vi "POO 1 - objet.vi"() -> ()   [LabVIEW 2023]
uses:
  Controller/Ctrl_ID.ctl
  Impot/Impot.lvclass
  ID/ID.lvclass
panel:
  in  "Annual ressource":dbl=100.0 format="%#_13g $"
  out "Tax evaluation":dbl
  out "Read ID after reset":T1
  out "Read ID":T1
  in  "Write ID":T1
  # "Write"
  # "Read"
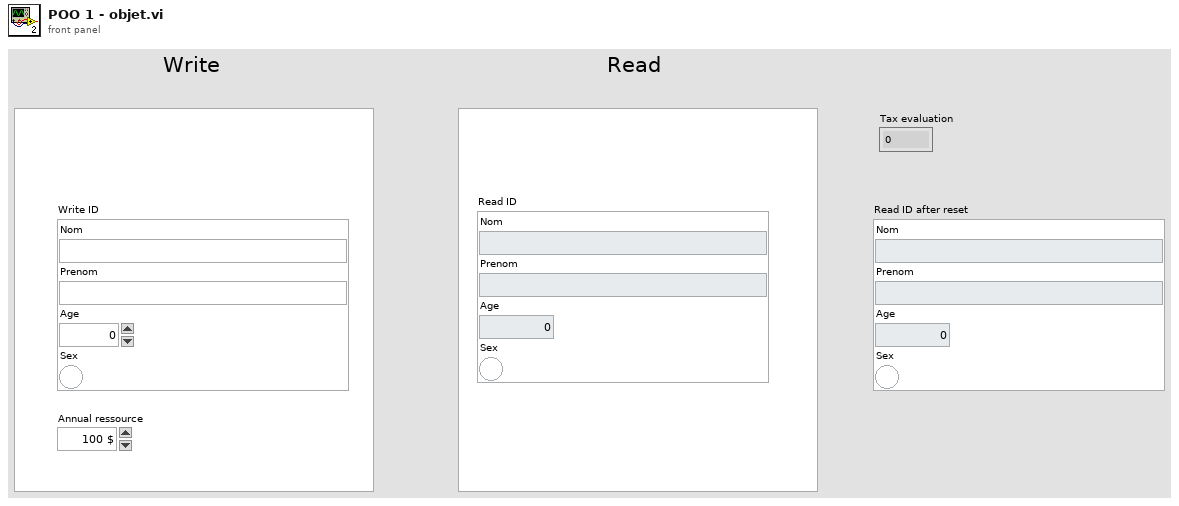
[diagram p1: front panel]
types:
  T1 = typedef "Ctrl_ID.ctl" = cluster{"Nom":string, "Prenom":string, "Age":u8, "Sex":bool}
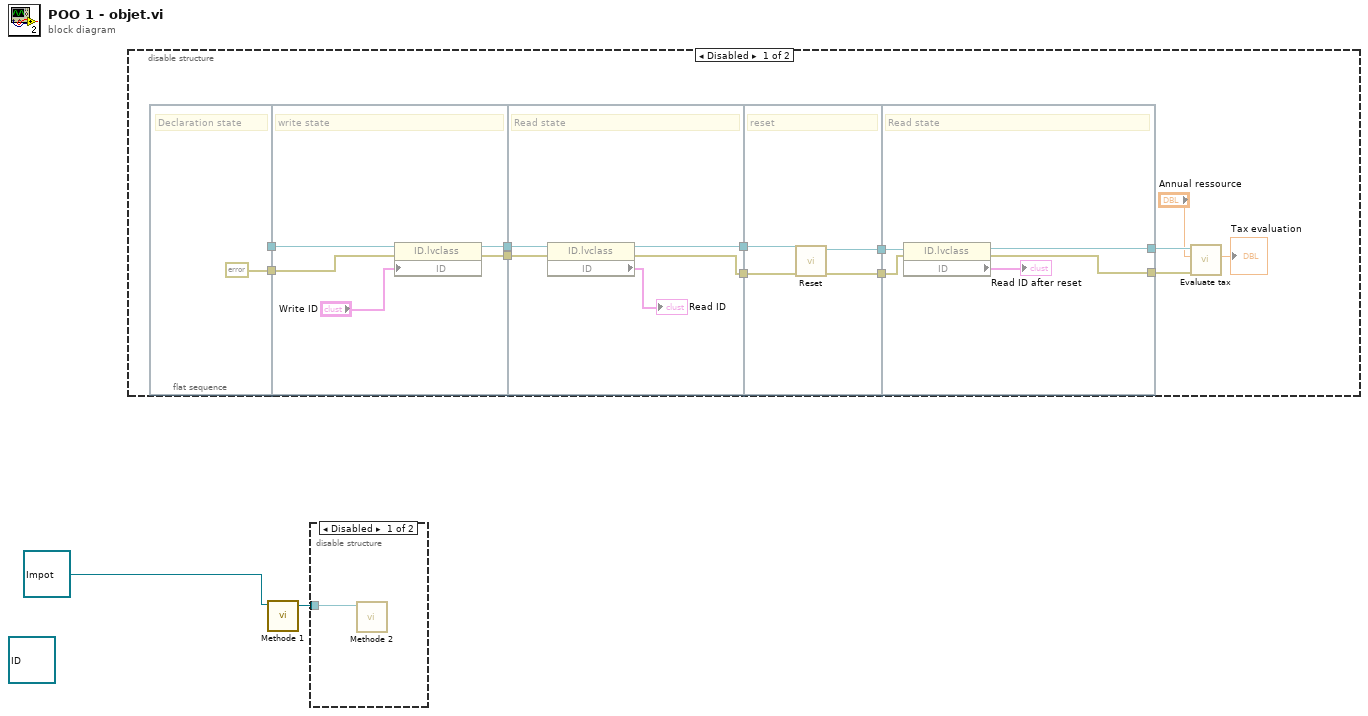
[diagram p0: block diagram]
diagram:
  (unwired) refnum<class "ID.lvclass"> refnum ("ID.lvclass")
  n1 = disable-structure shown="Disabled" {
    frame Disabled {
      n2 = flat-sequence {
        tunnel: [errorcluster {"status"=FALSE, "code"=0, "source"=""} ("error in (no error)")] -> w14
        tunnel: [_] -> w13
        tunnel: w14 -> [w18]
        tunnel: [w17] -> w12
        tunnel: [w16] -> w11
        tunnel: w13 -> [w20]
        tunnel: w12 -> [w24]
        tunnel: w11 -> [w25]
        tunnel: [w22] -> w10
        tunnel: [w21] -> w9
        tunnel: [w29] -> w8
        tunnel: [w28] -> w7
        tunnel: w10 -> [w27]
        tunnel: w9 -> [w26]
        tunnel: w8 -> [w33]
        tunnel: w7 -> [w34]
        tunnel: [w31] -> w6
        tunnel: [w30] -> w5
        frame #0 {
          # "Declaration state"
        }
        frame #1 {
          # "write state"
          n3 = property class="ID.lvclass"(reference=w20, error in=w18, "ID"="Write ID") -> (reference out=w17:refnum<class "ID.lvclass">, error out=w16:errorcluster)
        }
        frame #2 {
          # "Read state"
          n4 = property class="ID.lvclass"(reference=w24, error in=w25) -> (reference out=w22:refnum<class "ID.lvclass">, error out=w21:errorcluster, "ID"=→"Read ID":T1)
        }
        frame #3 {
          # "reset"
          n5 = call-dynamic "Reset.vi"("error in (no error)"=w26, "ID in"=w27) -> ("error out"=w29:errorcluster, "ID out"=w28:refnum<class "ID.lvclass">)  [unwired: 8 in]
        }
        frame #4 {
          # "Read state"
          n6 = property class="ID.lvclass"(reference=w34, error in=w33) -> (reference out=w31:refnum<class "ID.lvclass">, error out=w30:errorcluster, "ID"=→"Read ID after reset":T1)
        }
      }
      n7 = call "Evaluate tax.vi"("error in (no error)"=w5, "Annual ressource"="Annual ressource", "Impot in"=w6) -> ("Tax evaluation"=→"Tax evaluation":dbl)  [unwired: 6 in, 2 out]
    }
    frame Enabled {
    }
  }
  n8 = call "Methode 1.vi"("ID in"=refnum<class "Impot.lvclass"> refnum ("Impot.lvclass")) -> ("ID out"=w1:refnum<class "Impot.lvclass">)  [unwired: 9 in, 1 out]
  n9 = disable-structure shown="Disabled" {
    disable-tunnel: w1 -> [w35 _]
    frame Disabled {
      n10 = call "Methode 2.vi"("Impot in"=w35) -> ()  [unwired: 9 in, 2 out]
    }
    frame Enabled {
    }
  }
